vi "Cond Timed Wait (relative nanoseconds).vi"(8 "error in (no error)":errorcluster, 9 "relative timeout (nanoseconds)":i64, 10 "Mutex in":T1, 11 "Cond in":T2) -> (0 "error out":errorcluster, 1 "timed out?":bool, 2 "Mutex out":T1, 3 "Cond out":T2)   [LabVIEW 2013, in "POSIX Threads.lvlib" / "Cond.lvclass"]
uses:
  Cond.lvclass
  Controls/reference.ctl
  Mutex/Controls/reference.ctl
  Mutex/Mutex.lvclass
  Cond.lvclass/Cond.ctl
  POSIX Thread Object/POSIX Thread Object.lvclass/POSIX Thread Object.ctl
  POSIX Thread Object/Private VIs/libpthread path.vi
  <vilib>/NI/NI Linux RT Utilities/VIs/Public/Convert Types/convert timespec 64 to timespec 32.vi
  <vilib>/NI/NI Linux RT Utilities/VIs/Public/Time/Increment Time (timespec).vi
  <vilib>/NI/NI Linux RT Utilities/VIs/Public/Time/Get Clock Time (timespec).vi
  POSIX Thread Object/Private VIs/get pthread error.vi
  POSIX Thread Object/POSIX Thread Object.lvclass
  <vilib>/NI/NI Linux RT Utilities/Linux RT Utilities.lvlib
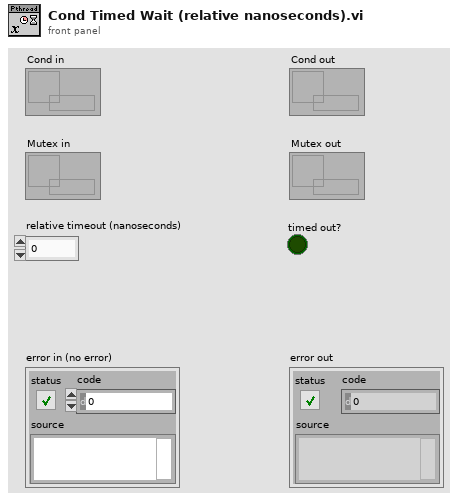
[diagram p1: front panel]
types:
  T1 = typedef "POSIX Threads.lvlib/Mutex.lvclass/reference.ctl" = refnum<data-value>
  T2 = typedef "POSIX Threads.lvlib/Cond.lvclass/reference.ctl" = refnum<data-value>
  T3 = typedef "Linux RT Utilities.lvlib/clockid_t.ctl" = enum16{"Realtime", "Monotonic"}
  T4 = typedef "Linux RT Utilities.lvlib/timespec_64.ctl" = cluster{"sec":u64, "nsec":u64}
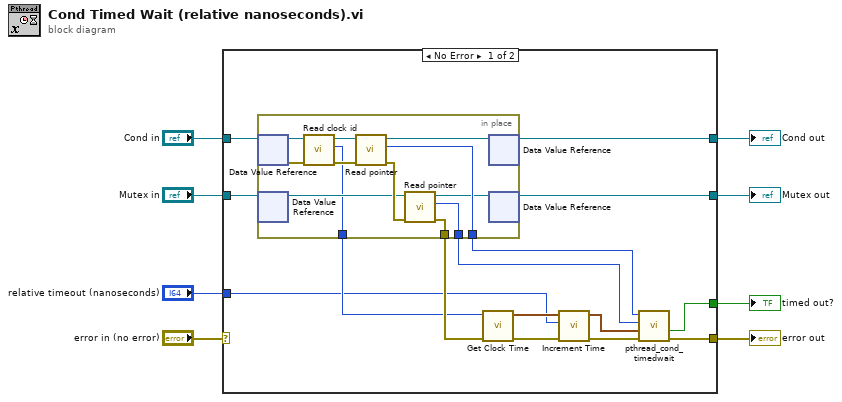
[diagram p0: block diagram]
diagram:
  n1 = case shown="No Error" "error in (no error)" {
    selector: "error in (no error)" -> [_ w38]
    tunnel: [w23 w38] -> w7
    tunnel: "Cond in" -> [w21 w37]
    tunnel: [w18 w37] -> w5
    tunnel: "Mutex in" -> [w20 w36]
    tunnel: [w17 w36] -> w3
    tunnel: "relative timeout (nanoseconds)" -> [w9 _]
    tunnel: [w22 _] -> w1
    frame No Error {
      n2 = in-place {
        in-place-border: [w34] -> w16
        in-place-border: [w32] -> w12
        in-place-border: [w31] -> w19
        in-place-border: [w24] -> w11
        n3 = in-place-dvr #1(w21) -> (w30:refnum<class "Cond.lvclass">, w29:errorcluster)
        n4 = in-place-dvr #2(w20) -> (w25:refnum<class "Mutex.lvclass">)  [unwired: 1 out]
        n5 = call "Read clock id.vi"("error in (no error)"=w29, "Cond in"=w30) -> ("error out"=w28:errorcluster, "lv_clockid_t"=w24:T3, "Cond out"=w27:refnum<class "Cond.lvclass">)  [unwired: 7 in]
        n6 = call "Read pointer.vi"("error in (no error)"=w28, "POSIX Thread Object in"=w27) -> ("error out"=w26:errorcluster, "pointer"=w34:u64, "POSIX Thread Object out"=w35:refnum<class "Cond.lvclass">)  [unwired: 7 in]
        n7 = call "Read pointer.vi"("error in (no error)"=w26, "POSIX Thread Object in"=w25) -> ("error out"=w32:errorcluster, "pointer"=w31:u64, "POSIX Thread Object out"=w33:refnum<class "Mutex.lvclass">)  [unwired: 7 in]
        n8 = in-place-dvr #1(w35) -> (w18:T2)  [unwired: 1 out]
        n9 = in-place-dvr #2(w33) -> (w17:T1)  [unwired: 1 out]
      }
      n10 = call-poly <vilib>:"Get Clock Time.vi"("error in (no error)"=w12, "clock id (monotonic)"=w11) -> ("error out"=w14:errorcluster, "timespec"=w10:T4)  [unwired: 8 in]
      n11 = call-poly <vilib>:"Increment Time.vi"("error in (no error)"=w14, "nanoseconds"=w9, "timespec in"=w10) -> ("error out"=w15:errorcluster, "timespec out"=w13:T4)  [unwired: 7 in]
      n12 = call "pthread_cond_timedwait.vi"("error in (no error)"=w15, "absolute time"=w13, "mutex ptr in"=w19, "cond ptr in"=w16) -> ("error out"=w23:errorcluster, "timed out?"=w22:bool)  [unwired: 4 in, 2 out]
    }
    frame Error {
    }
  }
  "Cond out" <- w5
  "error out" <- w7
  "Mutex out" <- w3
  "timed out?" <- w1
